vi "Actor Core.vi"(8 "error in":errorcluster, 11 "DataLog in":refnum<class "Template.lvclass">) -> (0 "error out":errorcluster, 3 "Actor out":refnum<class "Actor.lvclass">)   [LabVIEW 2020, in "Test Forms.lvlib" / "Template.lvclass"]
doc: "The user interface for this panel.\n\n----\nPlease see the following web address for additional documentation and tutorial information:\nhttp://www.mooregoodideas.com/mgi-panel-manager/\n\nAuthor: Derek Trepanier\n\nCopyright (c) 2018, Moore Good Ideas, Inc.\n\nAll rights reserved.\n\nRedistribution and use in source and binary forms, with or without modification, are permitted provided that the following conditions are met:\n\n * Redistributions of source code must retain the above copyright notice, this list of conditions and the following disclaimer.\n * Redistributions in binary form must reproduce the above copyright notice, this list of conditions and the following disclaimer in the documentation and/or other materials provided with the distribution.\n * Neither the name of Moore Good Ideas, Inc. nor the names of its contributors may be used to endorse or promote products derived from this software without specific prior written permission.\n\nTHIS SOFTWARE IS PROVIDED BY THE COPYRIGHT HOLDERS AND CONTRIBUTORS \"AS IS\" AND ANY EXPRESS OR IMPLIED WARRANTIES, INCLUDING, BUT NOT LIMITED TO, THE IMPLIED WARRANTIES OF MERCHANTABILITY AND FITNESS FOR A PARTICULAR PURPOSE ARE DISCLAIMED. IN NO EVENT SHALL THE COPYRIGHT OWNER OR CONTRIBUTORS BE LIABLE FOR ANY DIRECT, INDIRECT, INCIDENTAL, SPECIAL, EXEMPLARY, OR CONSEQUENTIAL DAMAGES (INCLUDING, BUT NOT LIMITED TO, PROCUREMENT OF SUBSTITUTE GOODS OR SERVICES; LOSS OF USE, DATA, OR PROFITS; OR BUSINESS INTERRUPTION) HOWEVER CAUSED AND ON ANY THEORY OF LIABILITY, WHETHER IN CONTRACT, STRICT LIABILITY, OR TORT (INCLUDING NEGLIGENCE OR OTHERWISE) ARISING IN ANY WAY OUT OF THE USE OF THIS SOFTWARE, EVEN IF ADVISED OF THE POSSIBILITY OF SUCH DAMAGE."
uses:
  Template.lvclass
  C:/Users/User/Desktop/Raman Program/LV-Database-OOP/source/Forms AF/Forms Controller/Form Controller/Panel Form Controller.lvclass
  <vilib>/ActorFramework/Actor/Actor.lvclass
  source/Forms AF/Forms Controller/Form Controller/Panel Form Controller.lvclass
  source/Forms AF/Forms Controller/Form Controller/Panel Form Controller.lvclass/Panel Form Controller.ctl
  source/Forms AF/Forms Controller/Open Form Button/Open Form Button.lvclass
  C:/Users/User/Desktop/Raman Program/LV-Database-OOP/source/Database OOP/Button Libraries/Button Interface Class/Button Interface.lvclass
  source/Database OOP/Column Libraries/Basic Field Constructors/Text Field.vi
  source/Forms AF/Forms Controller/Form Window/Form Window.lvclass
  source/Database OOP/Table Libraries/Basic Form/Basic Form.lvclass
  source/Database OOP/Column Libraries/Composed Field Constructors.lvlib
panel:
  in  "Numeric Field":dbl
  in  "Edit FK Ring":bool
  in  "String Field":string
  in  "FK Ring Field":u16(ring)
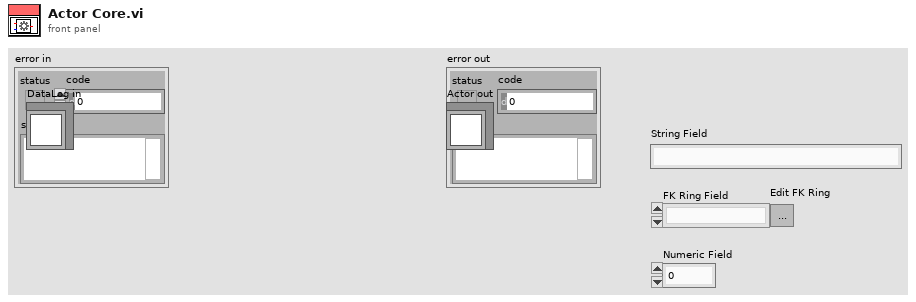
[diagram p1: front panel]
types:
  T1 = typedef "Panel Form Controller.lvlib/Builder Cluster.ctl" = cluster{"VI Ctrl Array":refnum<vi>[], "Form":refnum<class "Basic Form.lvclass">, "Open Form Button":refnum<class "Open Form Button.lvclass">}
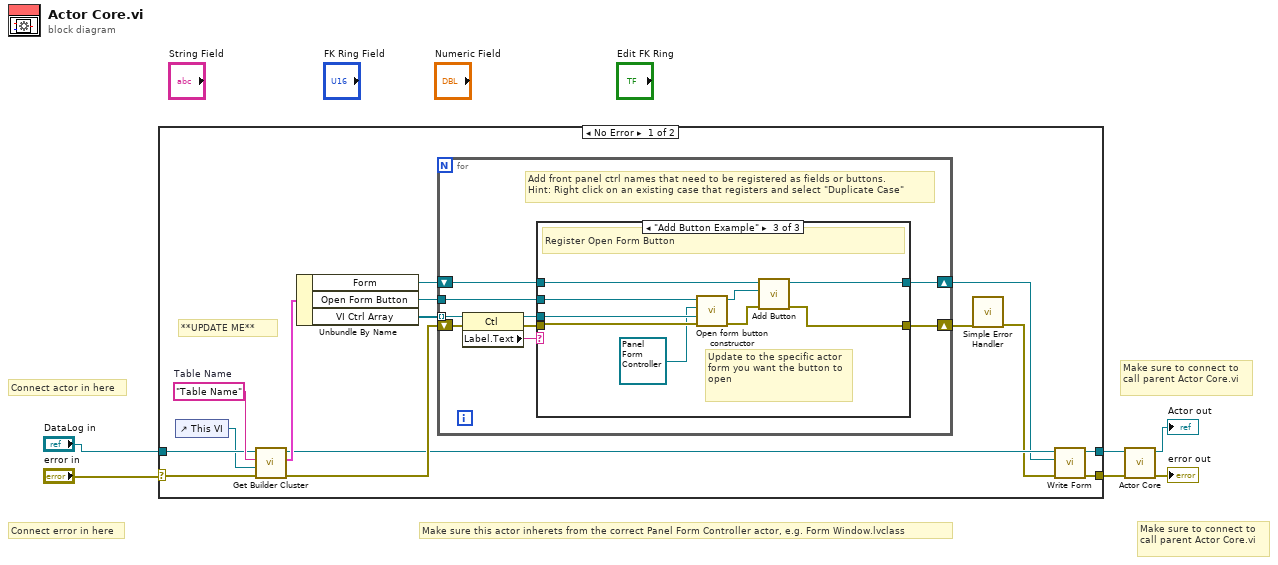
[diagram p0: block diagram]
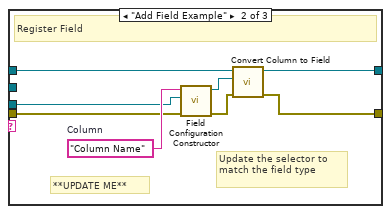
[diagram p3: hidden frame]
diagram:
  # "Make sure to connect to\ncall parent Actor Core.vi"
  # "Make sure to connect to\ncall parent Actor Core.vi"
  # "Make sure this actor inherets from the correct Panel Form Controller actor, e.g. Form Window.lvclass"
  # "Connect error in here"
  # "Connect actor in here"
  n1 = case shown="No Error" "error in" {
    selector: "error in" -> [w18 w51]
    tunnel: "DataLog in" -> [w8 w50]
    tunnel: [w12 w51] -> w3
    tunnel: [w13 w50] -> w4
    frame No Error {
      w11 = "Table Name"  # Table Name
      # "**UPDATE ME**"
      n2 = control-ref of="This VI"() -> (w7:refnum<vi>)
      n3 = call "Get Builder Cluster.vi"("error in (no error)"=w18, "VI Refnum"=w7, "Table Name"=w11, "Panel Form Controller in"=w8) -> ("error out"=w20:errorcluster, "Builder Cluster"=w19:T1, "Panel Form Controller out"=w15:refnum<class "Template.lvclass">)  [unwired: 5 in]
      n4 = Unbundle By Name(w19) -> ("Form"=w21:refnum<class "Basic Form.lvclass">, "Open Form Button"=w16:refnum<class "Open Form Button.lvclass">, "VI Ctrl Array"=w17:refnum<vi>[])
      n5 = for {
        tunnel: w17 -> [w30] mode=indexing
        shift-right: [w24] -> w14
        shift-left: w21 -> [w25]
        shift-right: [w22] -> w10
        shift-left: w20 -> [w28]
        tunnel: w16 -> [w23]
        # "Add front panel ctrl names that need to be registered as fields or buttons.\nHint: Right click on an existing case that registers and select \"Duplicate Case\""
        n6 = property class="Ctl"(reference=w30, error in=w28) -> (reference out=w29:refnum<vi>, error out=w27:errorcluster, "Label.Text"=w26:string)
        n7 = case shown="\"Add Button Example\"" w26 {
          tunnel: w29 -> [_ w35 w43]
          tunnel: w25 -> [w32 w40 w49]
          tunnel: [w32 w38 w48] -> w24
          tunnel: [w31 w39 w47] -> w22
          tunnel: w27 -> [w31 w34 w42]
          tunnel: w23 -> [_ _ w44]
          frame "", Default {
            # "Not Registered"
          }
          frame "Add Field Example" {
            w36 = "Column Name"  # Column
            # "Update the selector to match the field type"
            # "**UPDATE ME**"
            # "Register Field"
            n8 = call-poly "Field Configuration Constructor.vi"("error in"=w34, "Ctl Refnum"=w35, "Column Name"=w36) -> ("error out"=w37:errorcluster, "Field Configuration"=w33:refnum<class "Field Configuration.lvclass">)  [unwired: 7 in]
            n9 = call "Convert Column to Field.vi"("error in (no error)"=w37, "Field Configuration"=w33, "Basic Form in"=w40) -> ("error out"=w39:errorcluster, "Basic Form out"=w38:refnum<class "Basic Form.lvclass">)  [unwired: 7 in]
          }
          frame "Add Button Example" {
            # "Update to the specific actor form you want the button to open"
            # "Register Open Form Button"
            n10 = call "Open form button constructor.vi"("error in (no error)"=w42, "Ctl Refnum"=w43, "Panel Form"=refnum<class "Panel Form Controller.lvclass"> refnum ("Panel Form Controller.lvlib:Panel Form Controller.lvclass"), "Open Form Button in"=w44) -> ("error out"=w45:errorcluster, "Open Form Button out"=w46:refnum<class "Open Form Button.lvclass">)  [unwired: 6 in]
            n11 = call "Add Button.vi"("error in (no error)"=w45, "Button"=w46, "Basic Form in"=w49) -> ("error out"=w47:errorcluster, "Basic Form out"=w48:refnum<class "Basic Form.lvclass">)  [unwired: 7 in]
          }
        }
      }
      n12 = call <vilib>:"Simple Error Handler.vi"("error in (no error)"=w10) -> ("error out"=w9:errorcluster)  [unwired: 4 in, 4 out]
      n13 = call "Write Form.vi"("error in (no error)"=w9, "Form.lvlib:Basic Form.lvclass"=w14, "Panel Form Controller in"=w15) -> ("error out"=w12:errorcluster, "Panel Form Controller out"=w13:refnum<class "Template.lvclass">)  [unwired: 7 in]
    }
    frame Error {
    }
  }
  n14 = call-parent "Actor Core.vi"("error in"=w3, "Form Window in"=w4) -> ("error out"=→"error out":errorcluster, "Actor out"=→"Actor out":refnum<class "Actor.lvclass">)  [unwired: 8 in]
